vi "Fetch Analog Waveform.vi"(8 "error in (no error)":errorcluster, 9 "Timeout (10000 ms)":u32=10000, 10 "Source (0: Channel 1)":u16(ring) items=["Channel 1", "Channel 2", "Channel 3", "Channel 4", "Math"], 11 "VISA resource name":refnum<visa-resource-name>) -> (0 "error out":errorcluster, 2 "Waveform Data":waveform(dbl)(graph), 3 "VISA resource name out":refnum<visa-resource-name>)   [LabVIEW 2009, in "Agilent 6000 Series.lvlib"]
doc: "Returns the waveform the oscilloscope acquired for the specified channel. The waveform is from an acquisition that you initiate prior to calling this VI.\n\nYou use the Initiate VI to start an acquisition on the channels that you enable with the <B>Configure Channel</B> VI. The oscilloscope acquires waveforms for the enabled channels concurrently. You must call this VI separately for each enabled channel to obtain the waveforms.\n\nYou can call the <B>ag6000a Read Waveforms</B> VI instead of using low level VIs.\n\n<B>Note</B> This VI does not check the instrument status. Typically, you call this VI only in a sequence of calls to other low-level instrument driver VIs. The sequence performs one operation. You use the low-level VIs to optimize one or more aspects of interaction with the instrument."
uses:
  <instrlib>/Agilent 6000 Series/Agilent 6000 Series.lvlib
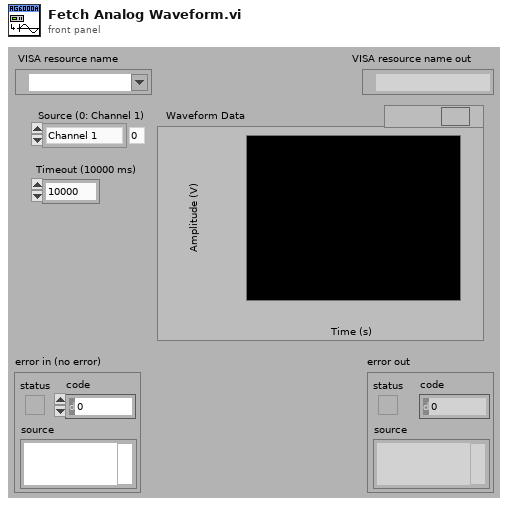
[diagram p1: front panel]
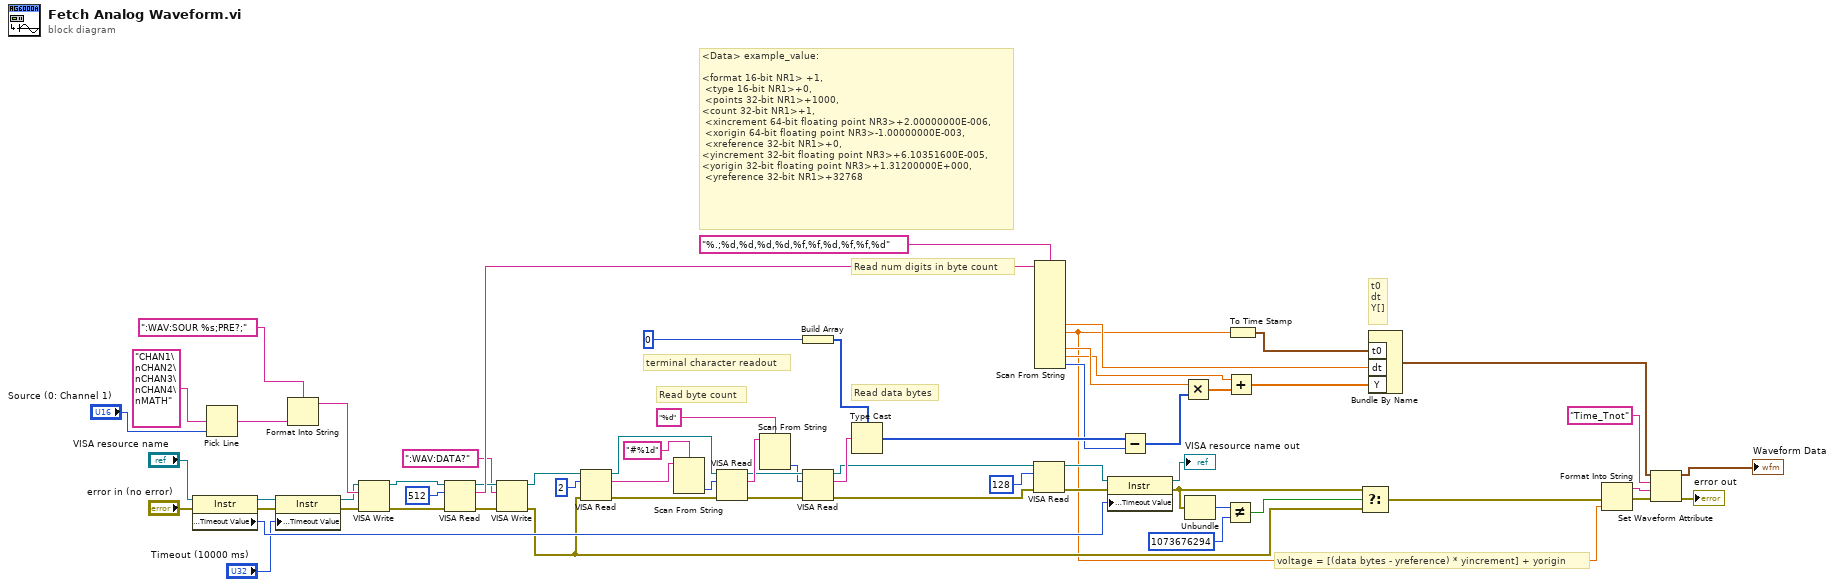
[diagram p0: block diagram]
diagram:
  # "voltage = [(data bytes - yreference) * yincrement] + yorigin"
  # "t0\ndt\nY[]"
  # "<Data> example_value:\n\n<format 16-bit NR1> +1,\n <type 16-bit NR1>+0,\n <points 32-bit NR1>+1000, \n<count 32-bit NR1>+1,\n <xincrement 64-bit floating point NR3>+2.00000000E-006,\n <xorigin 64-bit floating point NR3>-1.00000000E-003,\n <xreference 32-bit NR1>+0, \n<yincrement 32-bit floating point NR3>+6.10351600E-005, \n<yorigin 32-bit floating point NR3>+1.31200000E+000,\n <yreference 32-bit NR1>+32768"
  # "terminal character readout"
  # "Read data bytes"
  # "Read num digits in byte count"
  # "Read byte count"
  n1 = property on="Property Node" class="Instr"(reference="VISA resource name", error in="error in (no error)") -> (reference out=w49:refnum<visa-resource-name>, error out=w48:errorcluster, "General Settings:Timeout Value"=w50:u32)
  n2 = Pick Line(multi-line string="CHAN1\nCHAN2\nCHAN3\nCHAN4\nMATH", line index="Source (0: Channel 1)") -> (output string=w58:string)  [unwired: 1 in]
  n3 = property on="Property Node" class="Instr"(reference=w49, error in=w48, "General Settings:Timeout Value"="Timeout (10000 ms)") -> (reference out=w46:refnum<visa-resource-name>, error out=w45:errorcluster)
  n4 = Format Into String(format string=":WAV:SOUR %s;PRE?;", w58) -> (resulting string=w57:string)  [unwired: 2 in, 1 out]
  n5 = VISA Write(VISA resource name=w46, write buffer=w57, error in (no error)=w45) -> (VISA resource name out=w55:refnum<visa-resource-name>, error out=w56:errorcluster)  [unwired: 1 out]
  n6 = VISA Read(VISA resource name=w55, byte count=u32 512, error in (no error)=w56) -> (VISA resource name out=w44:refnum<visa-resource-name>, read buffer=w53:string, error out=w43:errorcluster)  [unwired: 1 out]
  n7 = VISA Write(VISA resource name=w44, write buffer=":WAV:DATA?", error in (no error)=w43) -> (VISA resource name out=w35:refnum<visa-resource-name>, error out=w18:errorcluster)  [unwired: 1 out]
  n8 = VISA Read(VISA resource name=w35, byte count=u32 2, error in (no error)=w18) -> (VISA resource name out=w38:refnum<visa-resource-name>, read buffer=w36:string, error out=w39:errorcluster)  [unwired: 1 out]
  n9 = Scan From String(format string="#%1d", input string=w36) -> (output 1=w37:i32)  [unwired: 3 in, 3 out]
  n10 = VISA Read(VISA resource name=w38, byte count=w37, error in (no error)=w39) -> (VISA resource name out=w31:refnum<visa-resource-name>, read buffer=w33:string, error out=w32:errorcluster)  [unwired: 1 out]
  n11 = Scan From String(format string="%d", input string=w33) -> (output 1=w29:i32)  [unwired: 3 in, 3 out]
  n12 = Build Array(u16 0) -> (w64:u16[])
  n13 = VISA Read(VISA resource name=w31, byte count=w29, error in (no error)=w32) -> (VISA resource name out=w27:refnum<visa-resource-name>, read buffer=w30:string, error out=w28:errorcluster)  [unwired: 1 out]
  n14 = Type Cast(type=w64, x=w30) -> (*(type *) &x=w14:u16[])
  n15 = VISA Read(VISA resource name=w27, byte count=u32 128, error in (no error)=w28) -> (VISA resource name out=w26:refnum<visa-resource-name>, error out=w25:errorcluster)  [unwired: 2 out]
  n16 = Scan From String(format string="%.;%d,%d,%d,%d,%f,%f,%d,%f,%f,%d", input string=w53) -> (output 5=w16:dbl, output 6=w3:dbl, output 8=w11:dbl, output 9=w9:dbl, output 10=w13:i32)  [unwired: 17 in, 3 out]
  n17 = property on="Property Node" class="Instr"(reference=w26, error in=w25, "General Settings:Timeout Value"=w50) -> (reference out=→"VISA resource name out":refnum<visa-resource-name>, error out=w20:errorcluster)
  n18 = Subtract(x=w14, y=w13) -> (x-y=w12:i32[])
  n19 = Multiply(x=w11, y=w12) -> (x*y=w10:dbl[])
  n20 = Unbundle(w20) -> ("code"=w23:i32)  [unwired: 2 out]
  n21 = Not Equal?(x=w23, y=1073676294) -> (x != y?=w21:bool)
  n22 = Add(x=w9, y=w10) -> (x+y=w15:dbl[])
  n23 = To Time Stamp(1:w3) -> (0:w17:timestamp)
  n24 = Select(t=w20, s=w21, f=w18) -> (s? t:f=w1:errorcluster)
  n25 = Bundle By Name ("Build Waveform")("t0"=w17, "dt"=w16, "Y"=w15) -> (w8:waveform(dbl))  [unwired: 1 in]
  n26 = Format Into String(error in=w1, w3) -> (resulting string=w4:string, error out=w2:errorcluster)  [unwired: 2 in]
  n27 = Set Waveform Attribute(4:w2, 5:w4, 6:"Time_Tnot" ("name"), 7:w8) -> (0:→"error out":errorcluster, 3:→"Waveform Data":waveform(dbl))  [unwired: 1 out]
